vi "Get RPM.vi"(8 "error in (no error)":errorcluster, 11 "Ismatech 3 Channel Settings In":T1={"VISA resource name"="", "Pump Number"=1, "Channel Number"=0, "Simulated?"=TRUE, "Reverse?"=FALSE} {"Channel Number" min=0 max=3; "Pump Number" min=1 max=9}) -> (0 "error out":errorcluster, 2 "RPM":dbl, 3 "Ismatech 3 Channel Settings Out":T1={"VISA resource name"="", "Pump Number"=1, "Channel Number"=0, "Simulated?"=TRUE, "Reverse?"=FALSE} {"Channel Number" min=0 max=3; "Pump Number" min=1 max=9})   [LabVIEW 2018, in "Ismatec 4308.lvlib"]
uses:
  Ismatec 4308.lvlib
  Ismatec 4083.ctl
  support/Support Library.lvlib
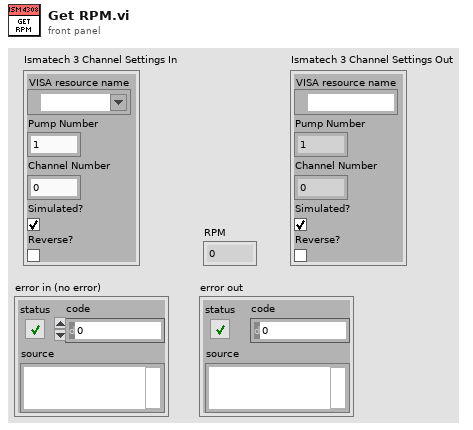
[diagram p1: front panel]
types:
  T1 = typedef "Ismatec 4308.lvlib/Ismatec 4083.ctl" = cluster{"VISA resource name":refnum<visa-resource-name>, "Pump Number":i16, "Channel Number":i16, "Simulated?":bool, "Reverse?":bool}
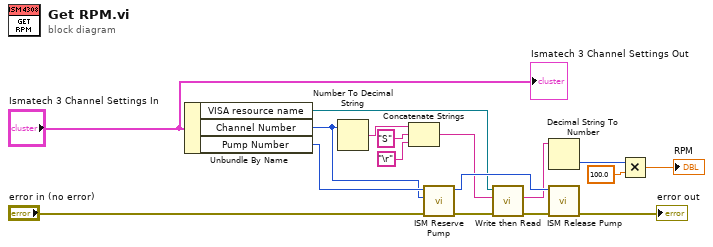
[diagram p0: block diagram]
diagram:
  n1 = Unbundle By Name("Ismatech 3 Channel Settings In") -> ("VISA resource name"=w6:refnum<visa-resource-name>, "Channel Number"=w1:i16, "Pump Number"=w7:i16)
  n2 = Number To Decimal String(number=w1) -> (decimal integer string=w12:string)  [unwired: 1 in]
  n3 = Concatenate Strings(w12, "S", "\r") -> (w5:string)
  n4 = call "ISM Reserve Pump.vi"("error in (no error)"="error in (no error)", "ISM Channel # In"=w1, "ISM Pump # In"=w7) -> ("error out"=w4:errorcluster, "ISM Pump # Out"=w10:i32)  [unwired: 7 in]
  n5 = call "Write then Read.vi"("error in"=w4, "write buffer"=w5, "VISA resource name in"=w6) -> ("error out"=w2:errorcluster, "read buffer"=w3:string)  [unwired: 6 in, 1 out]
  n6 = Decimal String To Number(string=w3) -> (number=w14:i32)  [unwired: 2 in, 1 out]
  n7 = call "ISM Release Pump.vi"("error in (no error)"=w2, "Pump Number In"=w10) -> ("error out"=→"error out":errorcluster)  [unwired: 8 in, 1 out]
  n8 = Multiply(x=w14, y=100.0) -> (x*y=→"RPM":dbl)
  "Ismatech 3 Channel Settings Out" <- "Ismatech 3 Channel Settings In"
